vi "Test - Check Event Structure Number.vi"() -> ()   [LabVIEW 2020]
uses:
  _csmHelper/API/Create From VI Reference.vi
  _csmHelper/API/Get Event Strucuture Num.vi
  _csmHelper/API/Check NewStateNotify is Registered.vi
  _csmHelper/API/Destroy.vi
  _csmHelper/CSM-Helper.lvclass
panel:
  out "NewStateNotify Registed":bool
  out "EvtStruNum":i32
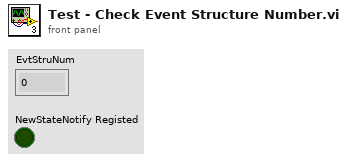
[diagram p1: front panel]
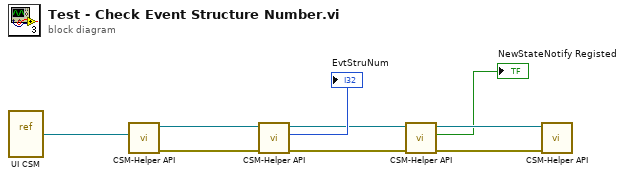
[diagram p0: block diagram]
diagram:
  n1 = vi-ref "UI CSM.vi"() -> (w9:refnum<vi>)
  n2 = call-poly "CSM-Helper API.vi"("VI"=w9) -> ("error out"=w7:errorcluster, "CSM-Helper.lvclass"=w8:refnum<class "CSM-Helper.lvclass">)  [unwired: 9 in]
  n3 = call-poly "CSM-Helper API.vi"("error in (no error)"=w7, "CSM-Helper in"=w8) -> ("error out"=w4:errorcluster, "EvtStruNum"=→"EvtStruNum":i32, "CSM-Helper out"=w5:refnum<class "CSM-Helper.lvclass">)  [unwired: 7 in]
  n4 = call-poly "CSM-Helper API.vi"("error in (no error)"=w4, "CSM-Helper in"=w5) -> ("error out"=w3:errorcluster, "NewStateNotify Registed"=→"NewStateNotify Registed":bool, "CSM-Helper out"=w2:refnum<class "CSM-Helper.lvclass">)  [unwired: 7 in]
  n5 = call-poly "CSM-Helper API.vi"("error in (no error)"=w3, "CSM-Helper in"=w2) -> ()  [unwired: 8 in, 2 out]
